vi "get_string.vi"(8 "error in (no error)":errorcluster, 11 "Mission in":refnum<class "Mission.lvclass">) -> (0 "error out":errorcluster, 2 "String":string, 3 "Mission out":refnum<class "Mission.lvclass">)   [LabVIEW 2011, in "Mission.lvclass"]
uses:
  Mission.lvclass
  Mission.lvclass/Mission.ctl
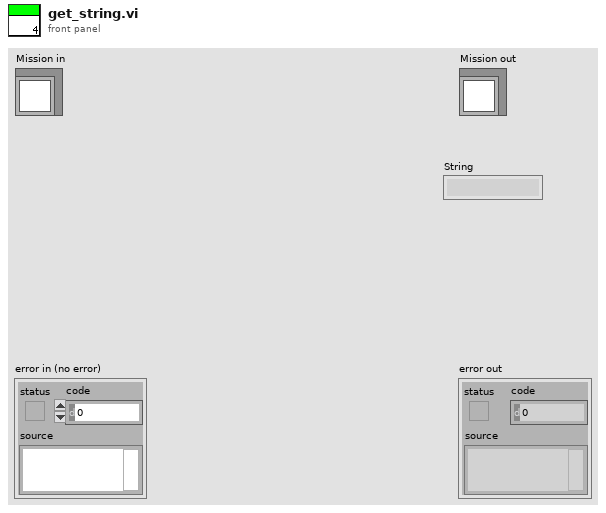
[diagram p1: front panel]
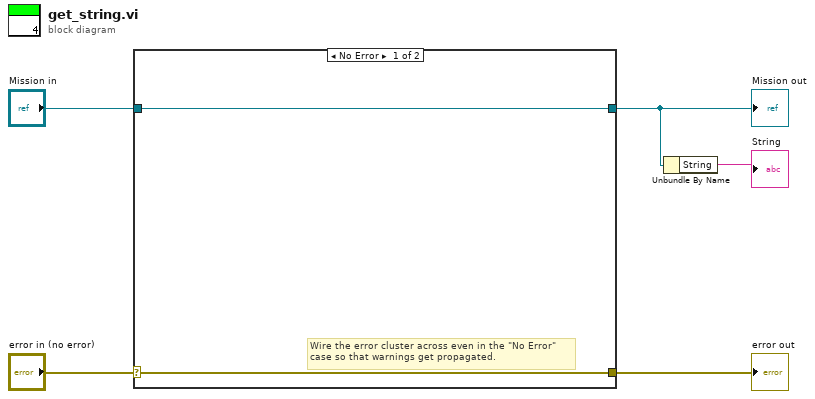
[diagram p0: block diagram]
diagram:
  n1 = case shown="No Error" "error in (no error)" {
    selector: "error in (no error)" -> [w6 w9]
    tunnel: [w6 w9] -> w4
    tunnel: [w7 w8] -> w2
    tunnel: "Mission in" -> [w7 w8]
    frame No Error {
      # "Wire the error cluster across even in the \"No Error\"\ncase so that warnings get propagated."
    }
    frame Error {
    }
  }
  "error out" <- w4
  "Mission out" <- w2
  n2 = Unbundle By Name(w2) -> ("String"=→"String":string)
